vi "Generated Descriptors.vi"() -> (3 "Descriptor Strings":string[](array[string]))   [LabVIEW 2021, in "Stream_server.lvlib"]
uses:
  Stream_server.lvlib
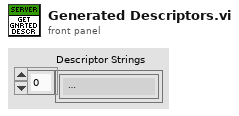
[diagram p1: front panel]
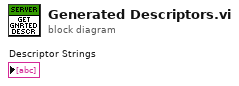
[diagram p0: block diagram]
diagram:
